vi "MatBuilder_Fill.vi"(9 "Columns":i32, 10 "Rows":i32, 11 "Value List":dbl[](array[numeric])) -> (3 "output matrix":T1)   [LabVIEW 2019, in "Trajectory_Library.lvlib"]
doc: "Fills the matrix with the given data, encoded in row major form. (The matrix is filled row by row, left to right with the given data).\n \nInputs:\n - Value List -- Array of values used to fill the matrix\n - Rows -- The number of rows in the resulting matrix\n - Columns -- The number of columns in the resulting matrix\n\nOutput:\n - Output Matrix -- The resulting filled matrix."
uses:
  Trajectory_Library.lvlib
  <vilib>/Analysis/Matrix/Datatypes/RealMatrix.ctl
  <vilib>/Analysis/Matrix/NI_Matrix.lvlib
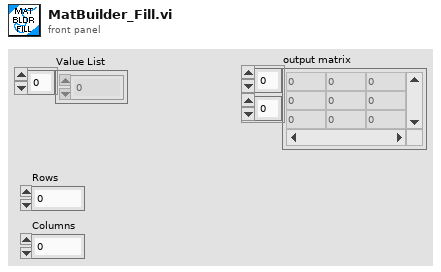
[diagram p1: front panel]
types:
  T1 = typedef "NI_Matrix.lvlib/RealMatrix.ctl" = dbl[][]
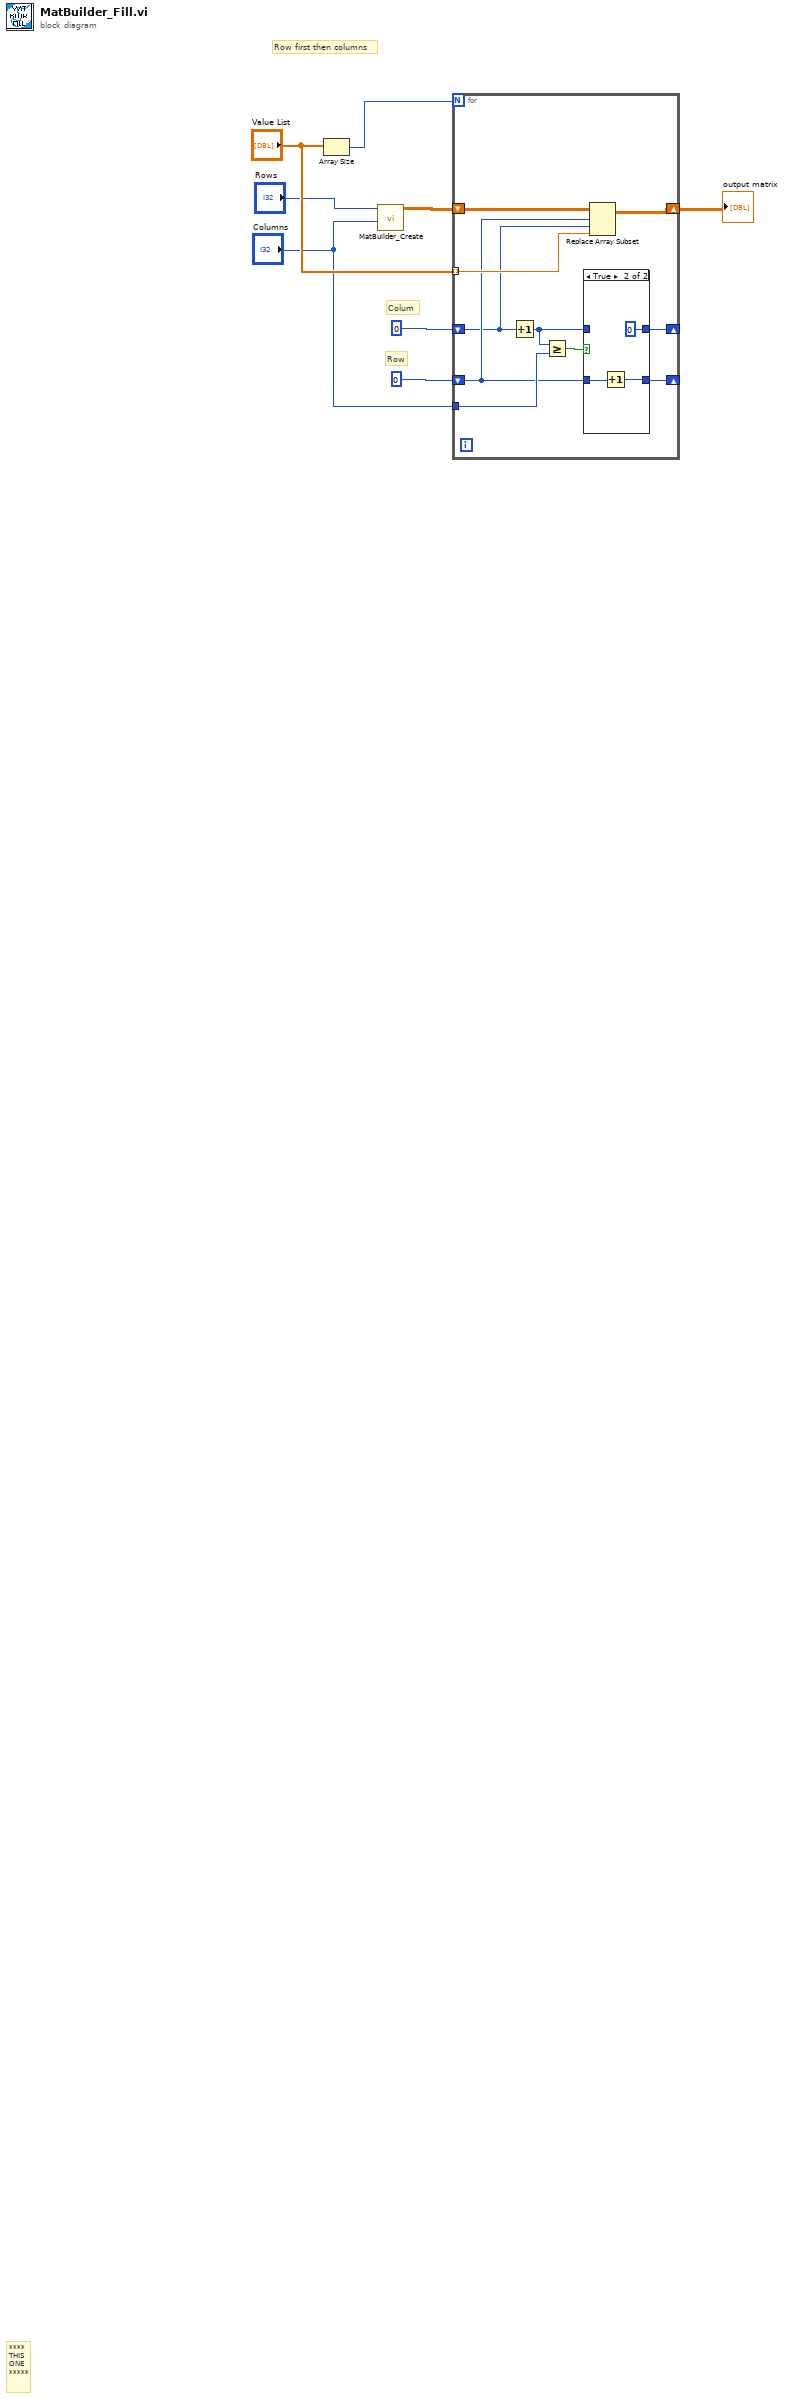
[diagram p0: block diagram]
diagram:
  # "Row first then columns"
  # "Row"
  # "Colum"
  # "****\nTHIS\nONE\n*****"
  n1 = Array Size(array="Value List") -> (size(s)=w8:i32)
  n2 = call "MatBuilder_Create.vi"("Columns"="Columns", "Rows"="Rows") -> ("output matrix"=w7:T1)  [unwired: 9 in]
  n3 = for {
    N: w8 -> [_]
    shift-right: [w16] -> w3
    shift-left: w7 -> [w18]
    tunnel: "Value List" -> [w17] mode=indexing
    tunnel: "Columns" -> [w13]
    shift-right: [w11] -> _
    shift-left: 0 -> [w9]
    shift-right: [w12] -> _
    shift-left: 0 -> [w10]
    n4 = Increment(x=w9) -> (x+1=w14:i32)
    n5 = Greater Or Equal?(x=w14, y=w13) -> (x >= y?=w15:bool)
    n6 = case shown="True" w15 {
      tunnel: w14 -> [w19 _]
      tunnel: w10 -> [w20 w23]
      tunnel: [w20 w22] -> w12
      tunnel: [w19 0] -> w11
      frame False {
      }
      frame True {
        n7 = Increment(x=w23) -> (x+1=w22:i32)
      }
    }
    n8 = Replace Array Subset(array=w18, new element=w17, index (row)=w10, index (col)=w9) -> (w16:T1)
  }
  "output matrix" <- w3
